vi "analysetemperature.vi"() -> ()   [LabVIEW 2013]
uses:
  <vilib>/Analysis/baseanly.llb/Mean (DBL).vi
  <vilib>/Analysis/NI_AALBase.lvlib
  <vilib>/Analysis/NI_AALPro.lvlib
panel:
  out "valeur min":dbl
  out "valeur max":dbl
  out "mean":dbl caption="moyenne" format="%0.2f"
  out "Graphe":cluster{dbl, i32, dbl[][]}(graph)
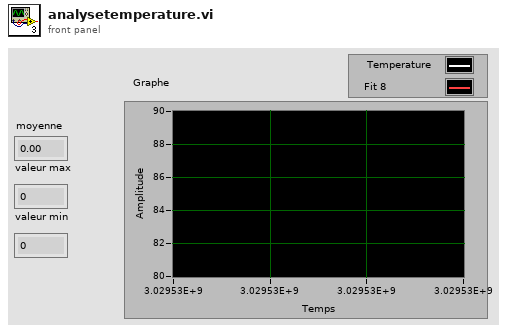
[diagram p1: front panel]
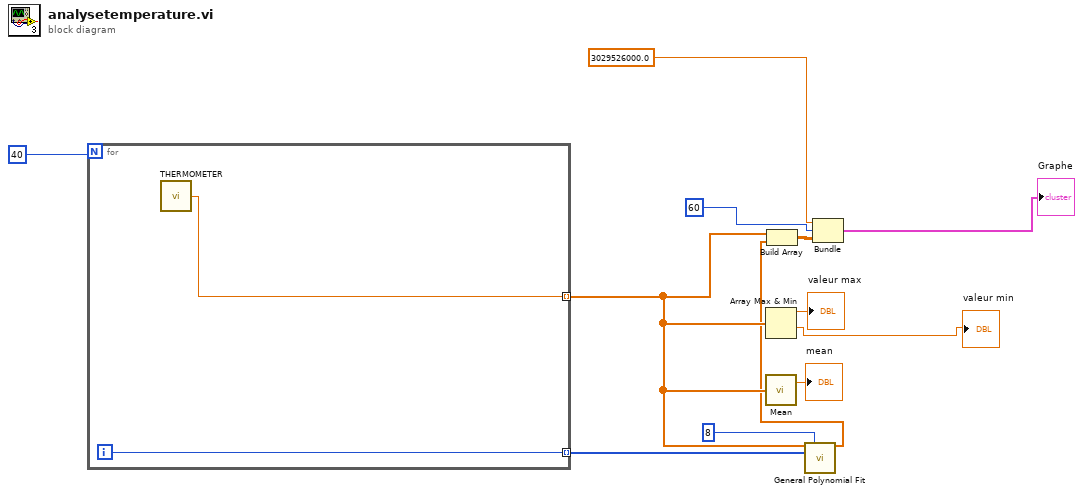
[diagram p0: block diagram]
diagram:
  n1 = for {
    N: 40 -> [_]
    tunnel: [w14] -> w4 mode=indexing
    tunnel: [w13] -> w5 mode=indexing
    i -> [w13]
    n2 = call "THERMOMETER.vi"() -> ("temeperature"=w14:dbl)  [unwired: 1 in]
  }
  n3 = Array Max & Min(array=w4) -> (max value=→"valeur max":dbl, min value=→"valeur min":dbl)  [unwired: 2 out]
  n4 = call-poly <vilib>:"Mean.vi"("X"=w4) -> ("mean"=→"mean":dbl)  [unwired: 1 out]
  n5 = call <vilib>:"General Polynomial Fit.vi"("Y"=w4, "polynomial order"=8, "X"=w5) -> ("Best Polynomial Fit"=w3:dbl[])  [unwired: 9 in, 3 out]
  n6 = Build Array(w4, w3) -> (w2:dbl[][])
  n7 = Bundle(3029526000.0, 60, w2) -> (→"Graphe":cluster{dbl, i32, dbl[][]})  [unwired: 1 in]
